vi "Global graph.vi"() -> ()   [LabVIEW 2013]
uses:
  Controls/Graph.ctl
panel:
  out "Dust Distribution":T1
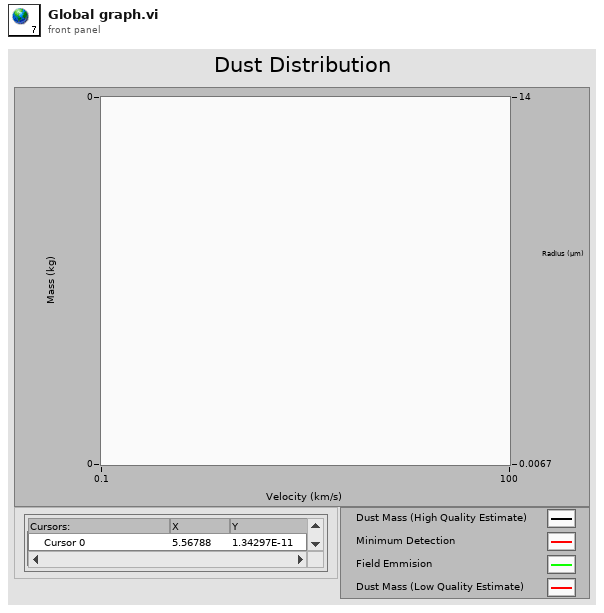
[diagram p1: front panel]
types:
  T1 = typedef "Graph.ctl" = cluster{cluster{"Vnoise":dbl, "Vnoise":dbl}[]}[]
diagram:
